vi "IOScan_InitWarnInfoControls.vi"(8 "error in":errorcluster, 11 "Scan Period Warn Info":T1) -> (0 "error out":errorcluster, 3 "Scan Period Warn Info out":T1)   [LabVIEW 2016]
uses:
  <resource>/dialog/TargetPreferencePages/IOScan_SubVIs/IOScan_PeriodWarnInfo.ctl
  <resource>/dialog/TargetPreferencePages/IOScan_SubVIs/IOScan_UIStrings.vi
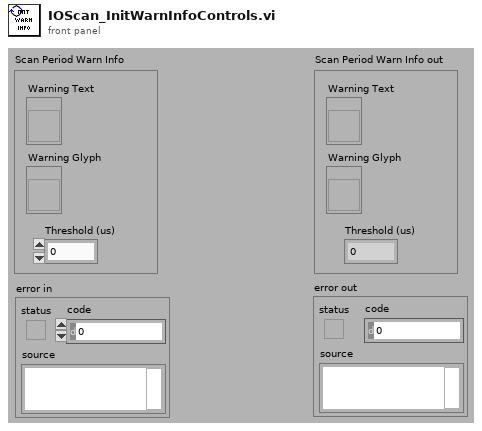
[diagram p1: front panel]
types:
  T1 = typedef "IOScan_PeriodWarnInfo.ctl" = cluster{"Warning Text":refnum<vi>, "Warning Glyph":refnum<vi>, "Threshold (us)":u32}
  T2 = enum8{"Enabled", "Disabled", "Disabled and Grayed Out"}
  T3 = typedef "IOScan_TimeUnit.ctl" = u16
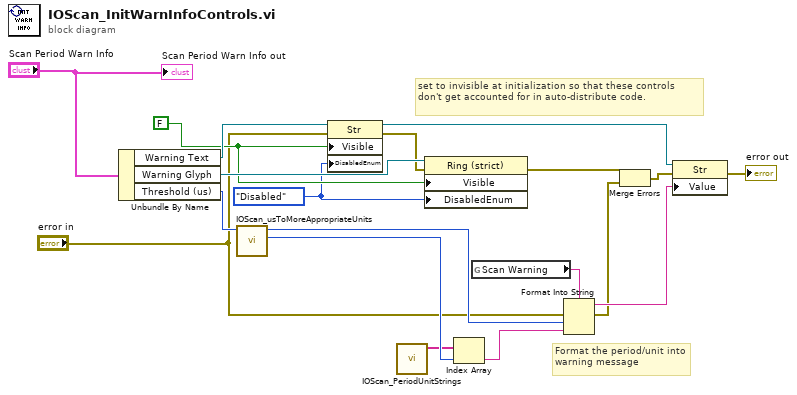
[diagram p0: block diagram]
diagram:
  w1 = T2."Disabled" ("Disabled")
  w5 = FALSE ("Visible")
  # "set to invisible at initialization so that these controls don't get accounted for in auto-distribute code."
  # "Format the period/unit into warning message"
  n1 = Unbundle By Name("Scan Period Warn Info") -> ("Warning Text"=w12:refnum<vi>, "Warning Glyph"=w11:refnum<vi>, "Threshold (us)"=w16:u32)
  n2 = call <resource>:"IOScan_usToMoreAppropriateUnits.vi"("Period (us)"=w16) -> ("Units"=w14:T3, "Period"=w15:u32)  [unwired: 8 in]
  n3 = property class="Str"(reference=w12, error in="error in", "Visible"=w5, "DisabledEnum"=w1) -> (reference out=w6:refnum<vi>, error out=w10:errorcluster)
  n4 = call <resource>:"IOScan_PeriodUnitStrings.vi"() -> ("Unit Strings"=w2:string[])  [unwired: 11 in]
  n5 = property class="Ring (strict)"(reference=w11, error in=w10, "Visible"=w5, "DisabledEnum"=w1) -> (error out=w9:errorcluster)  [unwired: 1 out]
  n6 = Index Array(array=w2, index=w14) -> (element=w13:string)
  n7 = global read "IOScan_UIStrings.vi" "Scan Warning"() -> (w4:string)
  n8 = Format Into String(format string=w4, error in="error in", w15, w13) -> (resulting string=w18:string, error out=w8:errorcluster)  [unwired: 1 in]
  n9 = Merge Errors(w9, w8) -> (w7:errorcluster)
  n10 = property class="Str"(reference=w6, error in=w7, "Value"=w18) -> (error out=→"error out":errorcluster)  [unwired: 1 out]
  "Scan Period Warn Info out" <- "Scan Period Warn Info"
